vi "Temperaturas.vi"() -> ()   [LabVIEW 2020]
panel:
  in  "Slide":dbl(slide) scale=0.0..100.0
  in  "?":bool
  out "Alarma":bool
  in  "Lim":dbl
  out "Grafico señal":dynamicdata(graph)
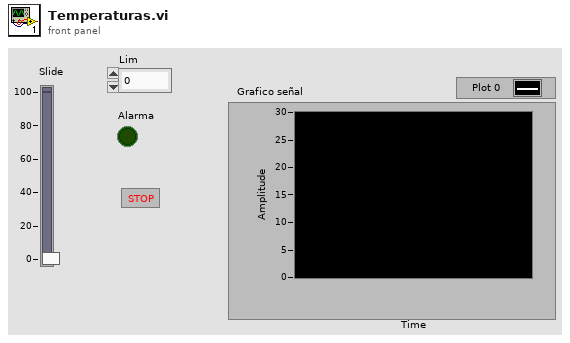
[diagram p1: front panel]
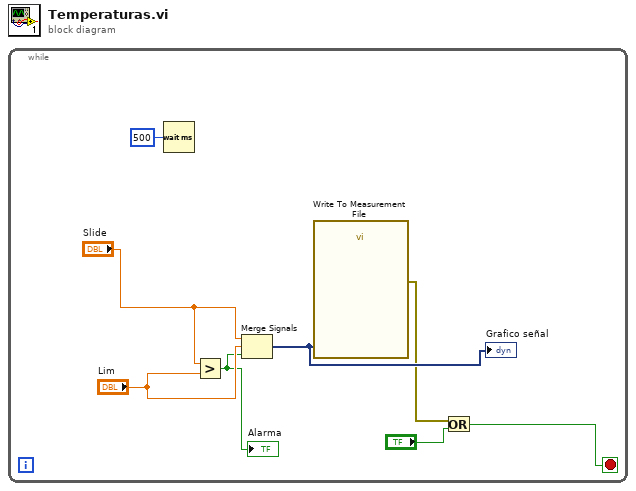
[diagram p0: block diagram]
diagram:
  n1 = while {
    stop <- w1 stop-if-true
    n2 = Wait (ms)(milliseconds to wait=u32 500) -> ()  [unwired: 1 out]
    n3 = Greater?(x="Slide", y="Lim") -> (0:w5:bool)
    "Alarma" <- w5
    n4 = Merge Signals("Slide", "Lim", w5) -> (w4:dynamicdata)
    "Grafico señal" <- w4
    n5 = call "Write To Measurement File"("Signals"=w4) -> ("error out"=w3:errorcluster)  [unwired: 16 in, 2 out]
    n6 = Or(x=w3, y="?") -> (x .or. y?=w1:bool)
  }
